vi "WriteToBaseConfigVariant.vi"(8 "error in (no error)":errorcluster, 10 "Variant":variant, 11 "ChromaAcLoad in":refnum<class "ChromaAcLoad.lvclass">) -> (0 "error out":errorcluster, 3 "ChromaAcLoad out":refnum<class "ChromaAcLoad.lvclass">)   [LabVIEW 2018, in "AcPwrPlugins.lvlib" / "ChromaAcLoad.lvclass"]
doc: "Write to the variant inside the base configuration."
uses:
  ChromaAcLoad.lvclass
  C:/Users/ico/Documents/Projects/NistPluggableModules/AcPwr/AcPwrPlugins/AcPwrBaseClass/AcPwrBase.lvclass
  AcPwrBaseClass/AcPwrBase.lvclass/AcPwrBase.ctl
  AcPwrBaseClass/Accessors/Read BaseConfig.vi
  AcPwrBaseClass/Accessors/Write BaseConfig.vi
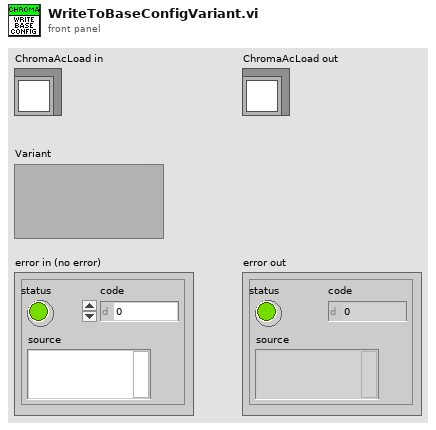
[diagram p1: front panel]
types:
  T1 = typedef "AcPwrPlugins.lvlib/AcPwrBase.lvclass/BaseConfig.ctl" = cluster{"Frequency":dbl, "FrequencyRange":dbl[], "Phases":T2[], "Name":string, "PPS":T3, "PluginConfigVariant":variant}
  T2 = typedef "AcPwrPlugins.lvlib/AcPwrBase.lvclass/Phase.ctl" = cluster{"Name":string, "Enabled":bool, "VoltageLevel":dbl, "Handle":string, "VoltageRange":dbl[], "Connected":bool, "CurrentLimit":dbl, "Waveform":string}
  T3 = typedef "AcPwrPlugins.lvlib/PacificPowerSource.lvclass/DeviceSettings.ctl" = cluster{"MeasName":string, "Modules":cluster{"Handle":string, "Connected":bool, "Clear Device (F)":bool, "btnIdQuery":bool, "btnReset":bool, "Program #":cluster{"Phase B (Degrees)":i32, "Waveform A (1: Sine)":i32, "Voltage Level (Va)":dbl, "Program Number (0)":i32, "Voltage Level (Vb) ":dbl, "Form (3: Three)":u16, "Coupling  (0: Direct)":u16, "Frequency (45Hz)":dbl, "Current Limit (40A)":dbl, "Phase C (Degrees)":i32, "Voltage Level (Vc)":dbl, "Waveform B (1: Sine)":i32, "Waveform C (1: Sine)":i32}[], "Impedance Parameters (off, 0.00)":cluster{"State":bool, "Impedance":dbl}, "Transient Execution (F)":bool, "OutputEnabled":bool, "Source Range":cluster{"Frequency Minimum (45 Hz)":dbl, "Frequency Maximum (1200 Hz)":dbl, "Voltage Maximum (V)":dbl, "Voltage Minimum (V)":dbl, "Range Control (0: Auto)":u16, "Initial Voltage (0V)":u16, "Frequency Range (600Hz)":u16}, "Port Type":enum16{"GPIB", "Serial"}}[]}
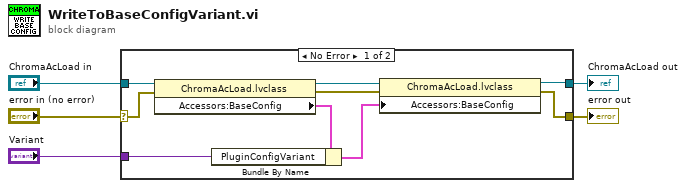
[diagram p0: block diagram]
diagram:
  n1 = case shown="No Error" "error in (no error)" {
    selector: "error in (no error)" -> [w13 w16]
    tunnel: [w9 w16] -> w4
    tunnel: [w7 w15] -> w2
    tunnel: "ChromaAcLoad in" -> [w14 w15]
    tunnel: "Variant" -> [w10 _]
    frame No Error {
      n2 = property class="ChromaAcLoad.lvclass"(reference=w14, error in=w13) -> (reference out=w8:refnum<class "ChromaAcLoad.lvclass">, error out=w12:errorcluster, "Accessors:BaseConfig"=w11:T1)
      n3 = Bundle By Name(cluster=w11, "PluginConfigVariant"=w10) -> (w6:T1)
      n4 = property class="ChromaAcLoad.lvclass"(reference=w8, error in=w12, "Accessors:BaseConfig"=w6) -> (reference out=w7:refnum<class "ChromaAcLoad.lvclass">, error out=w9:errorcluster)
    }
    frame Error {
    }
  }
  "error out" <- w4
  "ChromaAcLoad out" <- w2
